vi "SDG60RefClock.vi"(2 "error in (no error)":errorcluster, 3 "Ref 10MHz Src (T: Int)":bool=TRUE, 4 "10MHz Out (T:Enable)":bool=TRUE, 5 "VISA resource name":refnum<visa-resource-name>="USB0::0xF4EC::0x1101::SDG6XEBC5R0119::INSTR") -> (0 "error out":errorcluster, 1 "VISA resource name out":refnum<visa-resource-name>)   [LabVIEW 2018]
doc: "Configures the output impedance and source impedance for the channel you specify."
panel:
  # "If no valid external clock present,\noutputs will be switched off"
  # "Default state output state of\n10 MHz is off."
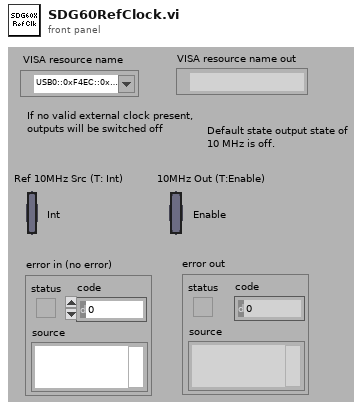
[diagram p1: front panel]
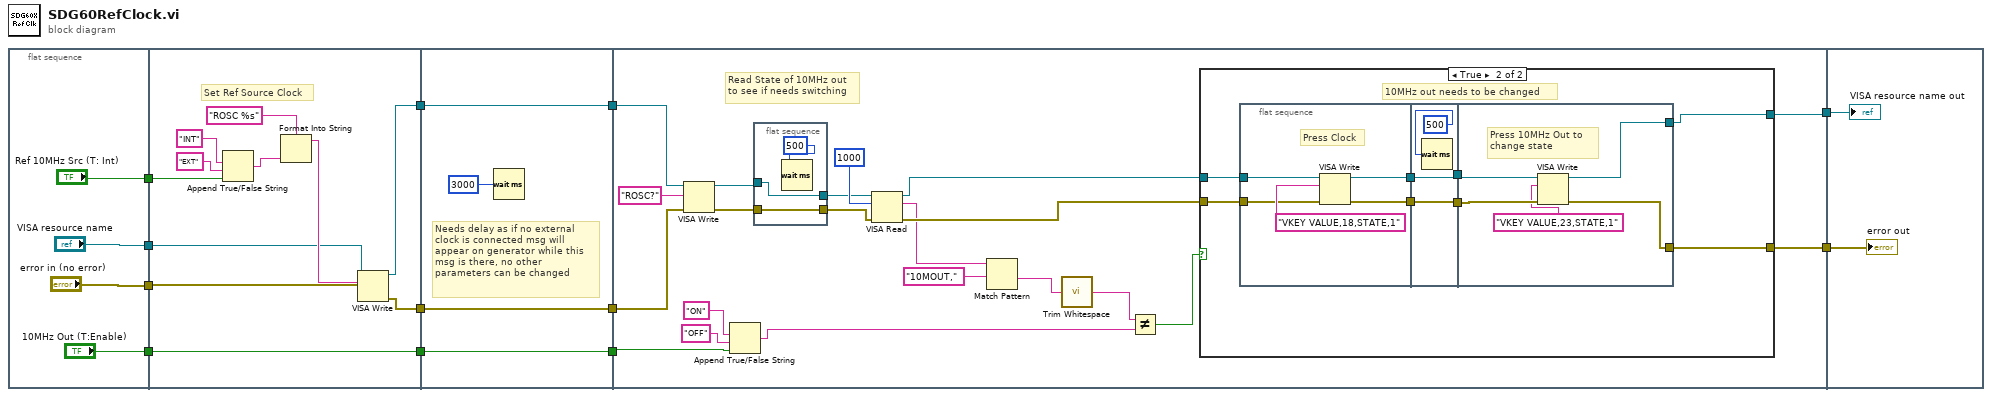
[diagram p0: block diagram]
diagram:
  n1 = flat-sequence {
    tunnel: ["Ref 10MHz Src (T: Int)"] -> w12
    tunnel: ["error in (no error)"] -> w11
    tunnel: ["VISA resource name"] -> w10
    tunnel: ["10MHz Out (T:Enable)"] -> w7
    tunnel: w12 -> [w22]
    tunnel: w11 -> [w21]
    tunnel: w10 -> [w20]
    tunnel: [w19] -> w6
    tunnel: [w18] -> w4
    tunnel: [w17] -> w2
    tunnel: w7 -> [w17]
    tunnel: w6 -> [w31]
    tunnel: [w31] -> w5
    tunnel: w4 -> [w30]
    tunnel: [w30] -> w3
    tunnel: w2 -> [w29]
    tunnel: [w29] -> w1
    tunnel: w5 -> [w48]
    tunnel: w3 -> [w47]
    tunnel: [w51] -> w9
    tunnel: [w52] -> w8
    tunnel: w1 -> [w38]
    tunnel: w9 -> [w79]
    tunnel: w8 -> [w80]
    frame #0 {
    }
    frame #1 {
      # "Set Ref Source Clock"
      n2 = Append True/False String(1:w22, 2:"EXT" ("true string"), 3:"INT" ("true string")) -> (0:w23:string)  [unwired: 1 in]
      n3 = Format Into String(format string="ROSC %s", w23) -> (resulting string=w24:string)  [unwired: 2 in, 1 out]
      n4 = VISA Write(VISA resource name=w20, write buffer=w24, error in (no error)=w21) -> (VISA resource name out=w19:refnum<visa-resource-name>, error out=w18:errorcluster)  [unwired: 1 out]
    }
    frame #2 {
      # "Needs delay as if no external \nclock is connected msg will \nappear on generator while this \nmsg is there, no other\nparameters can be changed"
      n5 = Wait (ms)(milliseconds to wait=3000) -> ()  [unwired: 1 out]
    }
    frame #3 {
      # "Read State of 10MHz out\nto see if needs switching"
      n6 = VISA Write(VISA resource name=w48, write buffer="ROSC?", error in (no error)=w47) -> (VISA resource name out=w46:refnum<visa-resource-name>, error out=w43:errorcluster)  [unwired: 1 out]
      n7 = Append True/False String(1:w38, 2:"OFF" ("true string"), 3:"ON" ("true string")) -> (0:w35:string)  [unwired: 1 in]
      n8 = flat-sequence {
        tunnel: w46 -> [w77]
        tunnel: [w77] -> w45
        tunnel: [w76] -> w44
        tunnel: w43 -> [w76]
        frame #0 {
          n9 = Wait (ms)(milliseconds to wait=500) -> ()  [unwired: 1 out]
        }
      }
      n10 = VISA Read(VISA resource name=w45, byte count=1000, error in (no error)=w44) -> (VISA resource name out=w41:refnum<visa-resource-name>, read buffer=w32:string, error out=w42:errorcluster)  [unwired: 1 out]
      n11 = Match Pattern(string=w32, regular expression="10MOUT,") -> (after substring=w34:string)  [unwired: 1 in, 3 out]
      n12 = call <vilib>:"Trim Whitespace.vi"("string"=w34) -> ("trimmed string"=w33:string)  [unwired: 1 in]
      n13 = Not Equal?(x=w33, y=w35) -> (x != y?=w36:bool)
      n14 = case shown="True" w36 {
        tunnel: [w54 w58] -> w52
        tunnel: [w53 w57] -> w51
        tunnel: w42 -> [w53 w56]
        tunnel: w41 -> [w54 w55]
        frame False {
          # "10MHz out doesn't need to be changed"
        }
        frame True {
          # "10MHz out needs to be changed"
          n15 = flat-sequence {
            tunnel: [w66] -> w62
            tunnel: [w65] -> w61
            tunnel: w56 -> [w64]
            tunnel: w55 -> [w63]
            tunnel: w62 -> [w69]
            tunnel: w61 -> [w68]
            tunnel: [w69] -> w60
            tunnel: [w68] -> w59
            tunnel: [w73] -> w57
            tunnel: [w72] -> w58
            tunnel: w60 -> [w75]
            tunnel: w59 -> [w74]
            frame #0 {
              # "Press Clock"
              n16 = VISA Write(VISA resource name=w63, write buffer="VKEY VALUE,18,STATE,1", error in (no error)=w64) -> (VISA resource name out=w66:refnum<visa-resource-name>, error out=w65:errorcluster)  [unwired: 1 out]
            }
            frame #1 {
              n17 = Wait (ms)(milliseconds to wait=500) -> ()  [unwired: 1 out]
            }
            frame #2 {
              # "Press 10MHz Out to \nchange state"
              n18 = VISA Write(VISA resource name=w75, write buffer="VKEY VALUE,23,STATE,1", error in (no error)=w74) -> (VISA resource name out=w72:refnum<visa-resource-name>, error out=w73:errorcluster)  [unwired: 1 out]
            }
          }
        }
      }
    }
    frame #4 {
      "error out" <- w79
      "VISA resource name out" <- w80
    }
  }
